vi "FinalChemProj.vi"() -> ()   [LabVIEW 2012]
uses:
  <userlib>/ImageProcessing/InitCamera_NTSC.vi
  <userlib>/ImageProcessing/FilterGreenPlane.vi
  <userlib>/ImageProcessing/FilterRedPlane.vi
panel:
  out "FoundElement":string
  out "Correct?":bool
  in  "?":bool
  out "Question":string
  out "SCORE":dbl
  out "Element":string[](array[string])
  out "x+y":dbl[](array[numeric])
  in  "Path":path=path "/Macintosh HD/Users/AswathyAshish/Desktop/FinalProj/Periodic table.csv"
  out "Periodic":string[][](array[string])
  out "Periodic Table":picture
  in  "Stop":bool
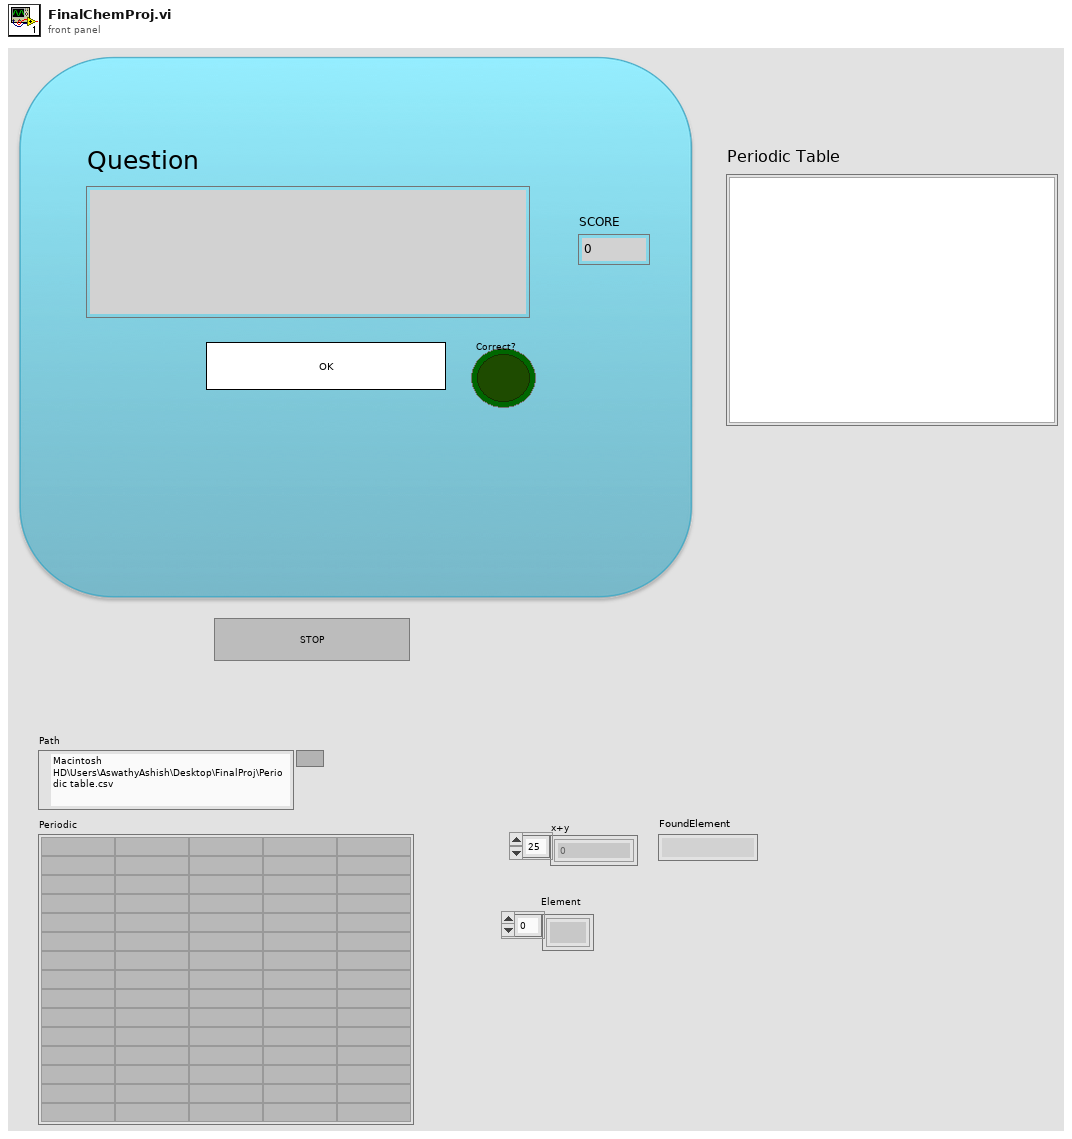
[diagram p1: front panel]
types:
  T1 = typedef "QT_Ref.ctl" = refnum<k1>
  T2 = cluster{"Width":u16, "Style":enum32{"Solid", "Dash", "Dot", "DashDot", "DashDotDot"}}
  T3 = typedef "QT_Image.ctl" = cluster{"Width":i32, "Height":i32, "Depth":i32, "data":u8[], "Compressed data":u8[], "Color table":u32[], "Duration":i32, "Options":i32, "Timestamp":i32, "ID":i32, "Reserved":i32, "Dialogs":u32}
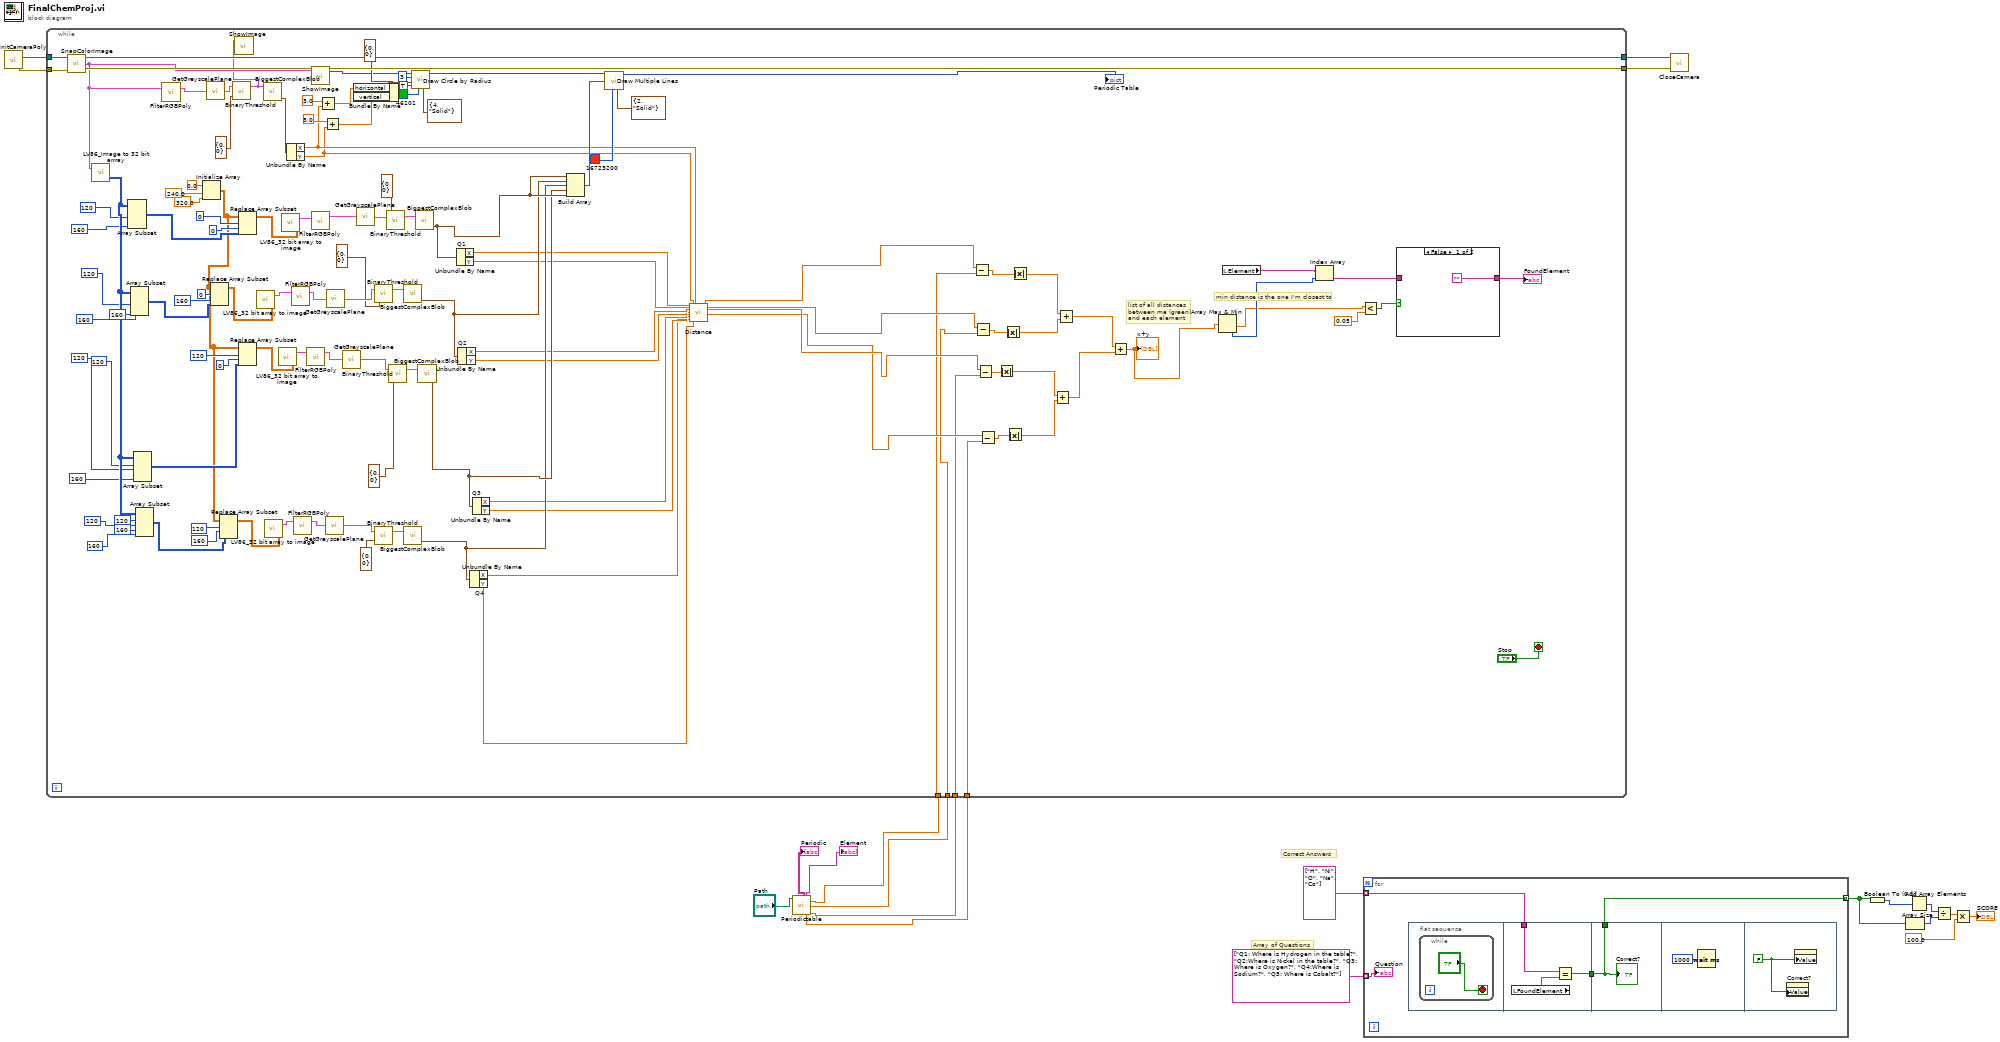
[diagram p0: block diagram]
diagram:
  # "Correct Answers"
  # "Array of Questions"
  n1 = call-poly <userlib>:"InitCameraPoly.vi"() -> ("error out"=w17:errorcluster, "QT Ref Out"=w18:T1)  [unwired: 2 in]
  n2 = call "Periodictable.vi"("Path"="Path") -> ("Periodic"=→"Periodic":string[][], "Element"=→"Element":string[], "Array 3"=w11:dbl[], "Array 6"=w14:dbl[], "Array 5"=w13:dbl[], "Array 4"=w12:dbl[])  [unwired: 9 in, 4 out]
  n3 = while {
    tunnel: w17 -> [w140]
    tunnel: w18 -> [w139]
    tunnel: [w138] -> w19
    tunnel: [w137] -> w20
    tunnel: w14 -> [w42]
    tunnel: w13 -> [w41]
    tunnel: w12 -> [w40]
    tunnel: w11 -> [w39]
    stop <- "Stop" stop-if-true
    # "min distance is the one I'm closest to"
    # "list of all distances\nbetween me (green)\nand each element"
    n4 = call <userlib>:"SnapColorImage.vi"("error in (no error)"=w140, "QT Ref In"=w139) -> ("error out"=w138:errorcluster, "Image Out"=w71:T3, "QT Ref Out"=w137:T1)  [unwired: 1 in]
    n5 = call <userlib>:"LV86_Image to 32 bit arrray.vi"("Image In"=w71) -> ("Intensity Graph"=w135:u32[][])  [unwired: 1 in, 1 out]
    n6 = Array Subset(array=w135, length (row)=120 ("length"), length (col)=160 ("length")) -> (w111:u32[][])  [unwired: 2 in]
    n7 = Array Subset(array=w135, length (row)=120 ("length"), index (col)=160 ("index"), length (col)=160 ("length")) -> (w122:u32[][])  [unwired: 1 in]
    n8 = Array Subset(array=w135, index (row)=120 ("index"), length (row)=120 ("length"), length (col)=160 ("length")) -> (w105:u32[][])  [unwired: 1 in]
    n9 = Array Subset(array=w135, index (row)=120 ("index"), length (row)=120 ("length"), index (col)=160 ("index"), length (col)=160 ("length")) -> (w102:u32[][])
    n10 = call-poly <userlib>:"FilterRGBPoly.vi"("Image in"=w71) -> ("Image out"=w74:T3)  [unwired: 1 in, 1 out]
    n11 = Initialize Array(0.0 ("element"), 240.0 ("element"), 320.0 ("element")) -> (w101:dbl[][])
    n12 = call <userlib>:"GetGreyscalePlane.vi"("Image In"=w74) -> ("Greyscale  Out"=w58:T3)
    n13 = Replace Array Subset(array=w101, new element=w122, index (row)=0, index (col)=160 ("index (row)")) -> (w121:dbl[][])
    n14 = Replace Array Subset(array=w101, new element=w102, index (row)=120, index (col)=160 ("index (row)")) -> (w99:dbl[][])
    n15 = call <userlib>:"BinaryThreshold.vi"("threshold"=cluster{u8, u8} {0, 0}, "Image In"=w58) -> ("Image Out"=w57:T3)  [unwired: 1 in]
    n16 = call <userlib>:"ShowImage.vi"("Image"=w57) -> ()  [unwired: 2 in, 2 out]
    n17 = Replace Array Subset(array=w101, new element=w111, index (row)=0, index (col)=0 ("index (row)")) -> (w110:dbl[][])
    n18 = Replace Array Subset(array=w101, new element=w105, index (row)=120, index (col)=0 ("index (row)")) -> (w100:dbl[][])
    n19 = call <userlib>:"LV86_32 bit array to image.vi"("Intensity Graph"=w121) -> ("Image Out"=w98:T3)  [unwired: 2 in]
    n20 = call <userlib>:"BiggestComplexBlob.vi"("Image in"=w57) -> ("Centroid"=w72:cluster{"X":dbl, "Y":dbl})  [unwired: 1 in, 2 out]
    n21 = call <userlib>:"LV86_32 bit array to image.vi"("Intensity Graph"=w99) -> ("Image Out"=w96:T3)  [unwired: 2 in]
    n22 = call <userlib>:"LV86_32 bit array to image.vi"("Intensity Graph"=w100) -> ("Image Out"=w97:T3)  [unwired: 2 in]
    n23 = call <userlib>:"LV86_32 bit array to image.vi"("Intensity Graph"=w110) -> ("Image Out"=w109:T3)  [unwired: 2 in]
    n24 = Unbundle By Name(w72) -> ("X"=w56:dbl, "Y"=w55:dbl)
    n25 = call-poly <userlib>:"FilterRGBPoly.vi"("Image in"=w98) -> ("Image out"=w95:T3)  [unwired: 1 in, 1 out]
    n26 = call-poly <userlib>:"FilterRGBPoly.vi"("Image in"=w96) -> ("Image out"=w93:T3)  [unwired: 1 in, 1 out]
    n27 = call-poly <userlib>:"FilterRGBPoly.vi"("Image in"=w97) -> ("Image out"=w94:T3)  [unwired: 1 in, 1 out]
    n28 = call <userlib>:"ShowImage.vi"("Image"=w71) -> ("image"=w59:picture)  [unwired: 2 in, 1 out]
    n29 = call-poly <userlib>:"FilterRGBPoly.vi"("Image in"=w109) -> ("Image out"=w108:T3)  [unwired: 1 in, 1 out]
    n30 = Add(x=3.0, y=w56) -> (x+y=w65:dbl)
    n31 = Add(x=3.0, y=w55) -> (x+y=w64:dbl)
    n32 = call <userlib>:"GetGreyscalePlane.vi"("Image In"=w93) -> ("Greyscale  Out"=w87:T3)
    n33 = call <userlib>:"GetGreyscalePlane.vi"("Image In"=w95) -> ("Greyscale  Out"=w89:T3)
    n34 = call <userlib>:"GetGreyscalePlane.vi"("Image In"=w94) -> ("Greyscale  Out"=w88:T3)
    n35 = Bundle By Name(cluster=cluster{"horizontal":i16, "vertical":i16} {"horizontal"=0, "vertical"=0} ("pixel center"), "horizontal"=w65, "vertical"=w64) -> (w69:cluster{"horizontal":i16, "vertical":i16})
    n36 = call <userlib>:"GetGreyscalePlane.vi"("Image In"=w108) -> ("Greyscale  Out"=w107:T3)
    n37 = call <userlib>:"BinaryThreshold.vi"("threshold"=cluster{u8, u8} {0, 0}, "Image In"=w89) -> ("Image Out"=w92:T3)  [unwired: 1 in]
    n38 = call <userlib>:"BinaryThreshold.vi"("threshold"=cluster{u8, u8} {0, 0}, "Image In"=w87) -> ("Image Out"=w90:T3)  [unwired: 1 in]
    n39 = call <userlib>:"BinaryThreshold.vi"("threshold"=cluster{u8, u8} {0, 0}, "Image In"=w107) -> ("Image Out"=w106:T3)  [unwired: 1 in]
    n40 = call <userlib>:"BinaryThreshold.vi"("threshold"=cluster{u8, u8} {0, 0}, "Image In"=w88) -> ("Image Out"=w91:T3)  [unwired: 1 in]
    n41 = call <userlib>:"BiggestComplexBlob.vi"("Image in"=w92) -> ("Centroid"=w77:cluster{"X":dbl, "Y":dbl})  [unwired: 1 in, 2 out]
    n42 = call <userlib>:"BiggestComplexBlob.vi"("Image in"=w90) -> ("Centroid"=w75:cluster{"X":dbl, "Y":dbl})  [unwired: 1 in, 2 out]
    n43 = call <vilib>:"Draw Circle by Radius.vi"("pen"=T2 {"Width"=4, "Style"=enum."Solid"}, "color(black)"=u32 46101, "fill?(F)"=TRUE, "pixel center"=w69, "radius"=i16 3, "picture"=w59) -> ("new picture"=w70:picture)  [unwired: 5 in]
    n44 = call <userlib>:"BiggestComplexBlob.vi"("Image in"=w106) -> ("Centroid"=w78:cluster{"X":dbl, "Y":dbl})  [unwired: 1 in, 2 out]
    n45 = call <userlib>:"BiggestComplexBlob.vi"("Image in"=w91) -> ("Centroid"=w76:cluster{"X":dbl, "Y":dbl})  [unwired: 1 in, 2 out]
    n46 = Unbundle By Name "Q1"(w78) -> ("X"=w54:dbl, "Y"=w53:dbl)
    n47 = Unbundle By Name "Q2"(w77) -> ("X"=w52:dbl, "Y"=w51:dbl)
    n48 = Unbundle By Name "Q4"(w75) -> ("X"=w48:dbl, "Y"=w47:dbl)
    n49 = Unbundle By Name "Q3"(w76) -> ("X"=w50:dbl, "Y"=w49:dbl)
    n50 = Build Array(w78, w77, w75, w76, w78) -> (w85:cluster{"X":dbl, "Y":dbl}[])
    n51 = call <vilib>:"Draw Multiple Lines.vi"("picture"=w70, "line endpoints"=w85, "color(black)"=u32 16723200, "pen"=T2 {"Width"=2, "Style"=enum."Solid"}) -> ("new picture"=→"Periodic Table":picture)  [unwired: 5 in]
    n52 = call "Distance.vi"("X1"=w54, "Y1"=w53, "X2"=w52, "Y2"=w51, "X3"=w50, "Y3"=w49, "x4"=w48, "Y"=w55, "Y4"=w47, "X"=w56) -> ("Ra1"=w46:dbl, "Ra2"=w45:dbl, "Ra3"=w44:dbl, "Ra4"=w43:dbl)  [unwired: 6 in, 8 out]
    n53 = Subtract(x=w46, y=w42) -> (x-y=w38:dbl[])
    n54 = Subtract(x=w45, y=w41) -> (x-y=w37:dbl[])
    n55 = Subtract(x=w44, y=w40) -> (x-y=w36:dbl[])
    n56 = Subtract(x=w43, y=w39) -> (x-y=w35:dbl[])
    n57 = Absolute Value(x=w36) -> (abs(x)=w32:dbl[])
    n58 = Absolute Value(x=w37) -> (abs(x)=w33:dbl[])
    n59 = Absolute Value(x=w35) -> (abs(x)=w31:dbl[])
    n60 = Absolute Value(x=w38) -> (abs(x)=w34:dbl[])
    n61 = Add(x=w32, y=w31) -> (x+y=w29:dbl[])
    n62 = Add(x=w34, y=w33) -> (x+y=w30:dbl[])
    n63 = Add(x=w30, y=w29) -> (x+y=w28:dbl[])
    "x+y" <- w28
    n64 = Array Max & Min(array=w28) -> (min value=w22:dbl, min index (indices)=w26:i32)  [unwired: 2 out]
    n65 = local read "Element"() -> (w27:string[])
    n66 = Index Array(array=w27, index=w26) -> (element=w25:string)
    n67 = Less?(x=w22, y=0.05) -> (x < y?=w23:bool)
    n68 = case shown="False" w23 {
      tunnel: w25 -> [_ w142]
      tunnel: ["" w142] -> w24
      frame False {
      }
      frame True {
      }
    }
    "FoundElement" <- w24
  }
  n69 = for {
    tunnel: string[] ["H", "Ni", "O", "Na", "Co"] -> [w145] mode=indexing
    tunnel: string[] ["Q1: Where is Hydrogen in the table?", "Q2:Where is Nickel in the table?", "Q3: Where is Oxygen?", "Q4:Where is Sodium?", "Q5: Where is Cobalt?"] -> [w146] mode=indexing
    tunnel: [w143] -> w2 mode=indexing
    n70 = flat-sequence {
      tunnel: w145 -> [w150]
      tunnel: [w149] -> w144
      tunnel: w144 -> [w151]
      tunnel: [w151] -> w143
      frame #0 {
        n71 = while {
          stop <- "?" stop-if-true
        }
      }
      frame #1 {
        n72 = local read "FoundElement"() -> (w148:string)
        n73 = Equal?(x=w150, y=w148) -> (x = y?=w149:bool)
      }
      frame #2 {
        "Correct?" <- w151
      }
      frame #3 {
        n74 = Wait (ms)(milliseconds to wait=u32 1000) -> ()  [unwired: 1 out]
      }
      frame #4 {
        w153 = FALSE
        n75 = property on="Correct?" class="Bool (strict)"("Value"=w153) -> ()  [unwired: 2 in, 2 out]
        n76 = property class="Bool (strict)"("Value"=w153) -> ()  [unwired: 2 in, 2 out]
      }
    }
    "Question" <- w146
  }
  n77 = call <userlib>:"CloseCamera.vi"("error in (no error)"=w19, "QT Ref In"=w20) -> ()  [unwired: 1 in, 1 out]
  n78 = Boolean To (0,1)(Boolean=w2) -> (0, 1=w9:i16[])
  n79 = Array Size(array=w2) -> (size(s)=w5:i32)
  n80 = Add Array Elements(numeric array=w9) -> (sum=w4:i16)
  n81 = Divide(x=w4, y=w5) -> (x/y=w6:dbl)
  n82 = Multiply(x=w6, y=100.0) -> (x*y=→"SCORE":dbl)
